vi "Double FFT Mesurament (Max Bin detection - Control - Init Wave&Window - Snapshot) RT Test.vi"() -> ()   [LabVIEW 2014]
uses:
  <vilib>/rvi/interface/nirviOpenFPGA/nirviOpenFPGA.xnode
  <vilib>/rvi/interface/nirviMethod/nirviMethod.xnode
  <vilib>/FPGAPlugInAG/Dynamic/niLvFpga_ConfigureFifo_Dynamic.vi
  <vilib>/rvi/errors/niLvFpgaMergeErrorWithErrorCode.vi
  <vilib>/FPGAPlugInAG/Dynamic/niLvFpga_StartFifo_Dynamic.vi
  <vilib>/FPGAPlugInAG/Dynamic/niLvFpga_Run_Dynamic.vi
  <vilib>/FPGAPlugInAG/Dynamic/niLvFpga_Abort_Dynamic.vi
  <vilib>/rvi/interface/nirviCloseFPGA/nirviCloseFPGA.xnode
  <vilib>/rvi/interface/nirviReadWriteControl/nirviReadWriteControl.xnode
  <vilib>/rvi/interface/Simulation/niFpgaSimulationCallBeginRW.vi
  <vilib>/rvi/errors/niLvFpgaAdjustHostInterfaceError.vi
  <vilib>/FPGAPlugInAG/Dynamic/niLvFpga_ReadFifo_Dynamic.vi
  NiFpgaLv.dll
  <vilib>/Utility/error.llb/Error Cluster From Error Code.vi
  <vilib>/Platform/TimedLoop/XDataNode/XDataNode.xnode
  <vilib>/Platform/TimedLoop/XDataNode/nitl_modes.ctl
  <vilib>/Platform/TimedLoop/XDataNode/XDNodeRunTimeDep.lvlib
  <vilib>/Platform/TimedLoop/XDataNode/wakeup.ctl
  <vilib>/Platform/TimedLoop/XDataNode/timing_clust.ctl
  <vilib>/FPGAPlugInAG/Dynamic/niLvFpga_Close_Dynamic.vi
  FPGA Target/Test VIs/Double FFT Mesurament (Max Bin detection - Control - Init Wave&Window - Snapshot) test.vi
panel:
  out "FFT (bin)":dbl[](graph)
  out "Signal (t)":waveform(dbl)(graph)
  in  "Snapshot":bool
  in  "Windowing":T1(ring)
  in  "first bin":i32=10
  in  "last bin":i32=255
  in  "lower limit 2":u32(slide)=677 scale=625.0..738.0
  in  "lower limit 1":u32(slide)=59 scale=0.0..113.0
  out "Detected Frequency Tone - (Hz)":dbl
  in  "stop":bool
  out "Max Bin":i32
  out "Max Amp":dbl format="%.2f"
  out "Prev Bin":i32
  out "Next Bin":i32
  out "Prev Amp":dbl format="%.2f"
  out "Next Amp":dbl format="%.2f"
  out "Interpolated Bin":dbl
  in  "Interpolation Method":T2(ring)=enum."Jain"
  # "WARNING:\nOnce pressed wait untill the end of operation"
  # "ONLINE parameter"
  # "OFFLINE parameters"
  # "Max Detection FFT bin range"
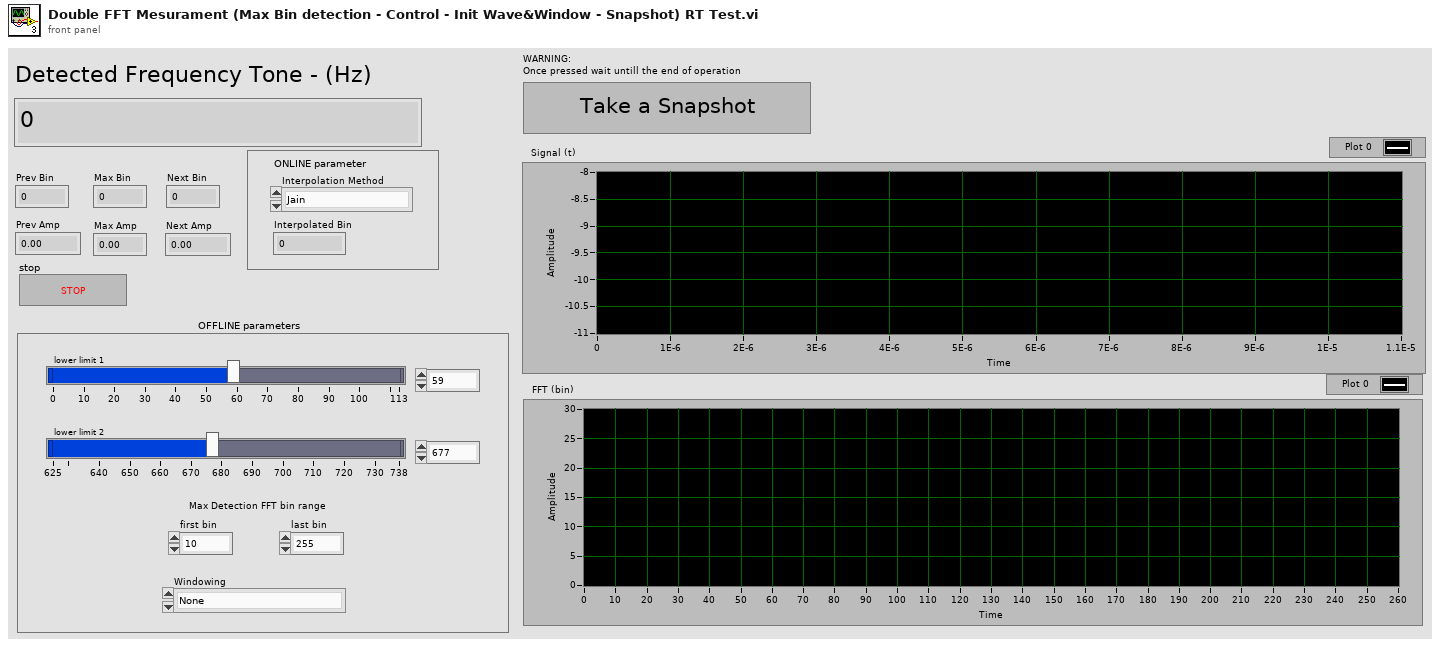
[diagram p1: front panel]
types:
  T1 = enum16{"None", "Hanning", "Hamming", "Blackman", "Blackman-Harris"}
  T2 = enum16{"Quadratic", "McLeodd", "Barycentric", "Jain"}
  T3 = typedef "XDNodeRunTimeDep.lvlib/timing_clust.ctl" = cluster{"Expected End [f-1]":u64, "Actual End [f-1]":u64, "Finished Late? [f-1]":bool, "Expected End [i-1]":u64, "Actual End [i-1]":u64, "Finished Late? [i-1]":bool, "Expected Start [i]":u64, "Actual Start [i]":u64, "Expected Start [f]":u64, "Actual Start [f]":u64, "Source Name":string, "Structure Name":string, "Period":i64, "Deadline":i64, "Offset":i64, "Start":i64, "Priority":i32, "Timeout":i32, "Mode":T4, "Wakeup Reason":T5, "Error":errorcluster, "Source Type":string, "Secondary Source Type":string, "Global End Time":u64, "Global Start Time":u64, "Frame Duration":u64, "Iteration Duration":u64, "Assigned CPU":i32, "I/O Scan Engine Mode":u32}
  T4 = typedef "XDNodeRunTimeDep.lvlib/nitl_modes.ctl" = enum32{"No Change", "Process missed periods, maintain original phase", "Discard missed periods, maintain original phase", "Process missed periods, ignore original phase", "Discard missed periods, ignore original phase"}
  T5 = typedef "XDNodeRunTimeDep.lvlib/wakeup.ctl" = enum32{"Normal", "Aborted", "Asynchronous wakeup", "Timing source error", "Timed loop error", "Timeout"}
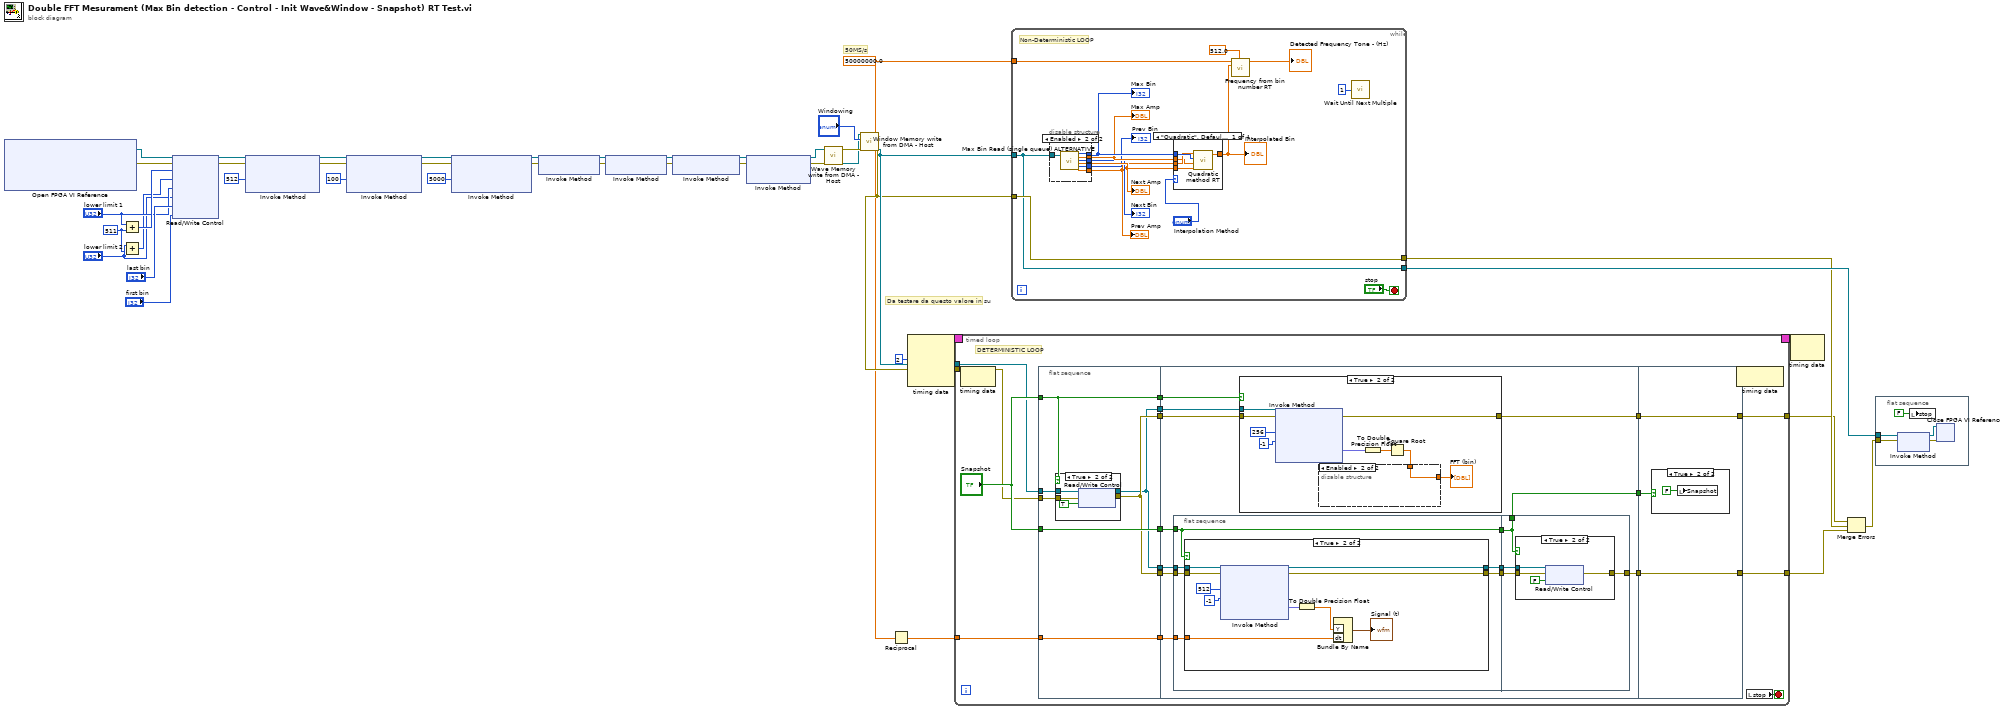
[diagram p0: block diagram]
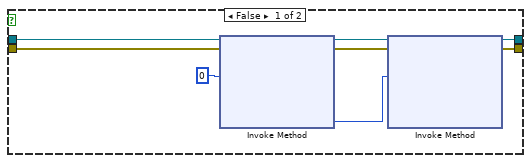
[diagram p3: hidden frame]
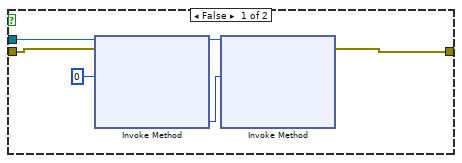
[diagram p5: hidden frame]
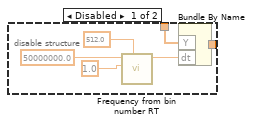
[diagram p6: hidden frame]
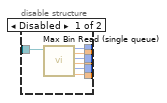
[diagram p8: hidden frame]
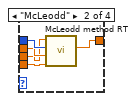
[diagram p9: hidden frame]
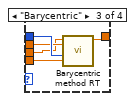
[diagram p10: hidden frame]
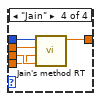
[diagram p11: hidden frame]
diagram:
  w37 = u32 511 ("y")
  w14 = 50000000.0 ("Sample Rate (S/s)")
  # "Da testare da questo valore in su"
  # "50MS/s"
  n1 = xnode "Open FPGA VI Reference"() -> ("FPGA VI Reference Out"=w36:refnum<k20>, "error out"=w35:errorcluster)  [unwired: 2 in]
  n2 = Add(x="lower limit 1", y=w37) -> (x+y=w41:u32)
  n3 = Add(x="lower limit 2", y=w37) -> (x+y=w39:u32)
  n4 = xnode "Read/Write Control"("FPGA VI Reference In"=w36, "error in"=w35, "upper limit 1"=w41, "upper limit 2"=w39, "lower limit 1"="lower limit 1", "lower limit 2"="lower limit 2", "last bin"="last bin", "first bin"="first bin") -> ("FPGA VI Reference Out"=w30:refnum<k20>, "error out"=w29:errorcluster)
  n5 = xnode "Invoke Method"("FPGA VI Reference In"=w30, "error in"=w29, "Requested Depth"=u32 512) -> ("FPGA VI Reference Out"=w28:refnum<k20>, "error out"=w27:errorcluster)  [unwired: 1 out]
  n6 = xnode "Invoke Method"("FPGA VI Reference In"=w28, "error in"=w27, "Requested Depth"=u32 100) -> ("FPGA VI Reference Out"=w26:refnum<k20>, "error out"=w25:errorcluster)  [unwired: 1 out]
  n7 = xnode "Invoke Method"("FPGA VI Reference In"=w26, "error in"=w25, "Requested Depth"=u32 5000) -> ("FPGA VI Reference Out"=w8:refnum<k20>, "error out"=w9:errorcluster)  [unwired: 1 out]
  n8 = xnode "Invoke Method"("FPGA VI Reference In"=w8, "error in"=w9) -> ("FPGA VI Reference Out"=w19:refnum<k20>, "error out"=w18:errorcluster)
  n9 = xnode "Invoke Method"("FPGA VI Reference In"=w19, "error in"=w18) -> ("FPGA VI Reference Out"=w21:refnum<k20>, "error out"=w20:errorcluster)
  n10 = xnode "Invoke Method"("FPGA VI Reference In"=w21, "error in"=w20) -> ("FPGA VI Reference Out"=w6:refnum<k20>, "error out"=w7:errorcluster)
  n11 = xnode "Invoke Method"("FPGA VI Reference In"=w6, "error in"=w7) -> ("FPGA VI Reference Out"=w13:refnum<k20>, "error out"=w12:errorcluster)  [unwired: 1 in]
  n12 = call "Wave Memory write from DMA - Host.vi"("error in"=w12, "FPGA VI Reference In"=w13) -> ("FPGA VI Reference Out"=w10:refnum<k20>, "error out"=w11:errorcluster)  [unwired: 7 in, 1 out]
  n13 = call "Window Memory write from DMA - Host.vi"("error in"=w11, "Enum"="Windowing", "FPGA VI Reference In"=w10) -> ("FPGA VI Reference Out"=w32:refnum<k20>, "error out"=w31:errorcluster)  [unwired: 5 in, 2 out]
  n14 = Reciprocal(x=w14) -> (1/x=w15:dbl)
  n15 = node-c288(i64 2 ("Period")) -> (w3:T3)  [unwired: 3 in]
  n16 = timed-loop {
    tunnel: w32 -> [w54]
    tunnel: w31 -> [w55]
    tunnel: [w57] -> w4
    tunnel: w15 -> [w59]
    tunnel: [w58] -> w5
    timing: w3 -> [_]
    timing-out: [_] -> w2
    stop <- w60 stop-if-true
    # "DETERMINISTIC LOOP"
    n17 = node-c288() -> ()  [unwired: 1 in, 1 out]
    n18 = flat-sequence {
      tunnel: w54 -> [w65]
      tunnel: w55 -> [w66]
      tunnel: "Snapshot" -> [w63]
      tunnel: "Snapshot" -> [w68]
      tunnel: w59 -> [w69]
      tunnel: [w67] -> w53
      tunnel: [w69] -> w52
      tunnel: [w68] -> w51
      tunnel: [w63] -> w50
      tunnel: [w67] -> w49
      tunnel: [w64] -> w48
      tunnel: [w64] -> w47
      tunnel: w53 -> [w85]
      tunnel: w52 -> [w84]
      tunnel: w51 -> [w77]
      tunnel: w50 -> [w81]
      tunnel: w49 -> [w80]
      tunnel: w48 -> [w79]
      tunnel: w47 -> [w86]
      tunnel: [w83] -> w46
      tunnel: [w82] -> w45
      tunnel: [w78] -> w44
      tunnel: [w146] -> w57
      tunnel: [w147] -> w58
      tunnel: w46 -> [w147]
      tunnel: w45 -> [w146]
      tunnel: w44 -> [w145]
      frame #0 {
        n19 = case shown="True" w63 {
          tunnel: [w70 w75] -> w67
          tunnel: w66 -> [w70 w74]
          tunnel: w65 -> [w71 w73]
          tunnel: [w71 w72] -> w64
          frame False {
          }
          frame True {
            n20 = xnode "Read/Write Control"("FPGA VI Reference In"=w73, "error in"=w74, "snapshot"=TRUE) -> ("FPGA VI Reference Out"=w72:refnum<k20>, "error out"=w75:errorcluster)
          }
        }
      }
      frame #1 {
        n21 = flat-sequence {
          tunnel: w86 -> [w95]
          tunnel: w85 -> [w94]
          tunnel: w84 -> [w93]
          tunnel: w77 -> [w90]
          tunnel: [w92] -> w89
          tunnel: [w91] -> w88
          tunnel: [w90] -> w87
          tunnel: [w115] -> w82
          tunnel: w89 -> [w117]
          tunnel: w88 -> [w116]
          tunnel: w87 -> [w114]
          tunnel: [w114] -> w78
          frame #0 {
            n22 = case shown="True" w90 {
              tunnel: w95 -> [w102 w113]
              tunnel: w94 -> [w100 w112]
              tunnel: [w99 w109] -> w91
              tunnel: w93 -> [_ w107]
              tunnel: [w96 w105] -> w92
              frame False {
                n23 = xnode "Invoke Method"("FPGA VI Reference In"=w102, "error in"=w100, "Number of Elements"=u32 0) -> ("FPGA VI Reference Out"=w98:refnum<k20>, "error out"=w97:errorcluster, "Elements Remaining"=w101:u32)  [unwired: 1 in, 1 out]
                n24 = xnode "Invoke Method"("FPGA VI Reference In"=w98, "error in"=w97, "Number of Elements"=w101) -> ("FPGA VI Reference Out"=w96:refnum<k20>, "error out"=w99:errorcluster)  [unwired: 1 in, 2 out]
              }
              frame True {
                n25 = xnode "Invoke Method"("FPGA VI Reference In"=w113, "error in"=w112, "Number of Elements"=u32 512, "Timeout (ms)"=-1) -> ("FPGA VI Reference Out"=w105:refnum<k20>, "error out"=w109:errorcluster, "Data"=w106:fxp<+/-,12,12>[])  [unwired: 1 out]
                n26 = To Double Precision Float(number=w106) -> (double precision float=w104:dbl[])
                n27 = Bundle By Name("Y"=w104, "dt"=w107) -> (→"Signal (t)":waveform(dbl))  [unwired: 1 in]
              }
            }
          }
          frame #1 {
            n28 = case shown="True" w114 {
              tunnel: [w118 w120] -> w115
              tunnel: w117 -> [_ w121]
              tunnel: w116 -> [w118 w119]
              frame False {
              }
              frame True {
                n29 = xnode "Read/Write Control"("FPGA VI Reference In"=w121, "error in"=w119, "snapshot"=FALSE) -> ("error out"=w120:errorcluster)  [unwired: 1 out]
              }
            }
          }
        }
        n30 = case shown="True" w81 {
          tunnel: w79 -> [w127 w129]
          tunnel: w80 -> [w124 w130]
          tunnel: [w123 w137] -> w83
          frame False {
            n31 = xnode "Invoke Method"("FPGA VI Reference In"=w127, "error in"=w124, "Number of Elements"=u32 0) -> ("FPGA VI Reference Out"=w125:refnum<k20>, "Elements Remaining"=w126:u32)  [unwired: 1 in, 2 out]
            n32 = xnode "Invoke Method"("FPGA VI Reference In"=w125, "Number of Elements"=w126) -> ("error out"=w123:errorcluster)  [unwired: 2 in, 3 out]
          }
          frame True {
            n33 = xnode "Invoke Method"("FPGA VI Reference In"=w129, "error in"=w130, "Number of Elements"=u32 256, "Timeout (ms)"=-1) -> ("error out"=w137:errorcluster, "Data"=w134:fxp<+,44,44>[])  [unwired: 2 out]
            n34 = To Double Precision Float(number=w134) -> (double precision float=w133:dbl[])
            n35 = Square Root(x=w133) -> (sqrt(x)=w132:dbl[])
            n36 = disable-structure shown="Enabled" {
              disable-tunnel: w132 -> [w139 w144]
              disable-tunnel: [w138 w144] -> w131
              frame Disabled {
                n37 = call "Frequency from bin number RT.vi"("FFT size"=512.0, "Bin number"=1.0, "Sample Rate (S/s)"=50000000.0) -> ("Detected Frequency (Hz)"=w140:dbl)  [unwired: 8 in]
                n38 = Bundle By Name("Y"=w139, "dt"=w140) -> (w138:waveform(dbl))  [unwired: 1 in]
              }
              frame Enabled {
              }
            }
            "FFT (bin)" <- w131
          }
        }
      }
      frame #2 {
        n39 = case shown="True" w145 {
          frame False {
          }
          frame True {
            n40 = local write "Snapshot"(FALSE ("Snapshot")) -> ()
          }
        }
      }
    }
    n41 = node-c288() -> ()  [unwired: 1 in, 1 out]
    n42 = local read "stop"() -> (w60:bool)
  }
  n43 = while {
    tunnel: w14 -> [w162]
    tunnel: w32 -> [w160]
    tunnel: w31 -> [w161]
    tunnel: [w160] -> w34
    tunnel: [w161] -> w17
    stop <- "stop" stop-if-true
    # "Non-Deterministic LOOP"
    n44 = disable-structure shown="Enabled" {
      disable-tunnel: w160 -> [w170 w177]
      disable-tunnel: [w169 w176] -> w156
      disable-tunnel: [w168 w175] -> w155
      disable-tunnel: [w167 w173] -> w154
      disable-tunnel: [w166 w171] -> w153
      disable-tunnel: [w165 w172] -> w152
      disable-tunnel: [w164 w174] -> w151
      frame Disabled {
        n45 = call "Max Bin Read (single queue).vi"("FPGA VI Reference In"=w170) -> ("Max Bin"=w169:i32, "Max Amp"=w168:dbl, "Next Bin"=w164:i32, "Next Amp"=w167:dbl, "Prev Bin"=w165:i32, "Prev Amp"=w166:dbl)  [unwired: 13 in]
      }
      frame Enabled {
        n46 = call "Max Bin Read (single queue) ALTERNATIVE.vi"("FPGA VI Reference In"=w177) -> ("Max Bin"=w176:i32, "Max Amp"=w175:dbl, "Next Bin"=w174:i32, "Next Amp"=w173:dbl, "Prev Bin"=w172:i32, "Prev Amp"=w171:dbl)  [unwired: 13 in]
      }
    }
    "Max Bin" <- w156
    "Max Amp" <- w155
    "Prev Bin" <- w152
    "Next Bin" <- w151
    "Prev Amp" <- w153
    "Next Amp" <- w154
    n47 = case shown="\"Quadratic\", Default" "Interpolation Method" {
      tunnel: w156 -> [w181 w186 w191 w196]
      tunnel: w155 -> [w178 w185 w190 w195]
      tunnel: w153 -> [w179 w184 w189 w194]
      tunnel: w154 -> [w180 w183 w188 w193]
      tunnel: [w182 w187 w192 w197] -> w157
      frame "Quadratic", Default {
        n48 = call "Quadratic method RT.vi"("Next Amplitude"=w180, "Max Amplitude"=w178, "Max bin"=w181, "Prev Amplitude"=w179) -> ("Bin"=w182:dbl)  [unwired: 7 in]
      }
      frame "McLeodd" {
        n49 = call "McLeodd method RT.vi"("Next Amp"=w183, "Max Amp"=w185, "Max Bin"=w186, "Prev Amp"=w184) -> ("Bin"=w187:dbl)  [unwired: 7 in]
      }
      frame "Barycentric" {
        n50 = call "Barycentric method RT.vi"("Next Amp"=w188, "Max Bin"=w191, "Max Amp"=w190, "Prev Amp"=w189) -> ("Bin"=w192:dbl)  [unwired: 7 in]
      }
      frame "Jain" {
        n51 = call "Jain's method RT.vi"("Prev Amp"=w194, "Next Amp"=w193, "Max Amp"=w195, "Max Bin"=w196) -> ("Bin"=w197:dbl)  [unwired: 7 in]
      }
    }
    "Interpolated Bin" <- w157
    n52 = call "Frequency from bin number RT.vi"("FFT size"=512.0, "Bin number"=w157, "Sample Rate (S/s)"=w162) -> ("Detected Frequency (Hz)"=→"Detected Frequency Tone - (Hz)":dbl)  [unwired: 8 in]
    n53 = call "Wait Until Next Multiple"("Count(mSec)"=u32 1 ("Count(uSec)")) -> ()  [unwired: 1 out]
  }
  n54 = node-c288(w2) -> ()  [unwired: 1 out]
  n55 = Merge Errors(w5, w17, w4) -> (w16:errorcluster)
  n56 = flat-sequence {
    tunnel: w34 -> [w200]
    tunnel: w16 -> [w199]
    frame #0 {
      n57 = xnode "Invoke Method"("FPGA VI Reference In"=w200, "error in"=w199) -> ("FPGA VI Reference Out"=w201:refnum<k20>, "error out"=w202:errorcluster)
      n58 = local write "stop"(FALSE ("stop")) -> ()
      n59 = xnode "Close FPGA VI Reference"("FPGA VI Reference In"=w201, "error in"=w202) -> ()  [unwired: 1 out]
    }
  }
